vi "set output trigger type.vi"(8 "error in (no error)":errorcluster, 10 "Output trigger connector":T1=enum."3", 11 "DAQOrcaFlash in":refnum<class "DAQOrcaFlash.lvclass">) -> (0 "error out":errorcluster, 3 "DAQOrcaFlash out":refnum<class "DAQOrcaFlash.lvclass">)   [LabVIEW 2012, in "DAQOrcaFlash.lvclass"]
uses:
  DAQOrcaFlash.lvclass
  connector.ctl
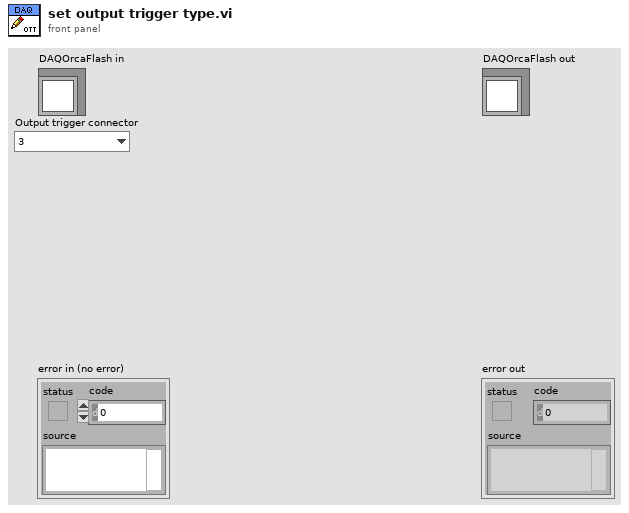
[diagram p1: front panel]
types:
  T1 = typedef "DAQOrcaFlash.lvclass/connector.ctl" = enum32{"1", "2", "3"}
  T2 = typedef "DAQOrcaFlash.lvclass/output trigger type.ctl" = sgl
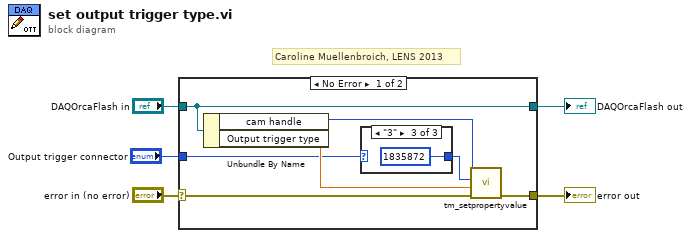
[diagram p0: block diagram]
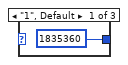
[diagram p2: hidden frame]
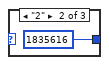
[diagram p3: hidden frame]
diagram:
  # "Caroline Muellenbroich, LENS 2013"
  n1 = case shown="No Error" "error in (no error)" {
    selector: "error in (no error)" -> [w11 w17]
    tunnel: [w10 w17] -> w4
    tunnel: [w12 w16] -> w2
    tunnel: "DAQOrcaFlash in" -> [w12 w16]
    tunnel: "Output trigger connector" -> [w6 _]
    frame No Error {
      n2 = Unbundle By Name(w12) -> ("cam handle"=w9:u32, "Output trigger type"=w7:T2)
      n3 = case shown="\"3\"" w6 {
        tunnel: [u32 1835360 ("Property ID") u32 1835616 ("Property ID") u32 1835872 ("Property ID")] -> w8
        frame "1", Default {
        }
        frame "2" {
        }
        frame "3" {
        }
      }
      n4 = call <userlib>:"tm_setpropertyvalue.vi"("error in (no error)"=w11, "Value in"=w7, "Property ID"=w8, "Handle in"=w9) -> ("error out"=w10:errorcluster)  [unwired: 6 in, 1 out]
    }
    frame Error {
    }
  }
  "error out" <- w4
  "DAQOrcaFlash out" <- w2
